vi "SR430.ProcEvents.vi"(0 "i ref in":refnum<vi>, 5 "error in (no error)":errorcluster) -> (14 "i ref out":refnum<vi>, 19 "error out":errorcluster)   [LabVIEW 2014, in "SR430.lvlib"]
doc: "Definition of commands for this class."
uses:
  SR430.lvlib
  CSCore/BaseProcess/BaseProcess.event definition.ctl
  CSCore/CAEObj/CAEObj.event definition.ctl
  CSCore/BaseProcess/BaseProcess.descriptor string definition.ctl
  CSCore/BaseProcess/BaseProcess.lvlib
  CSCore/CAEObj/CAEObj.lvlib
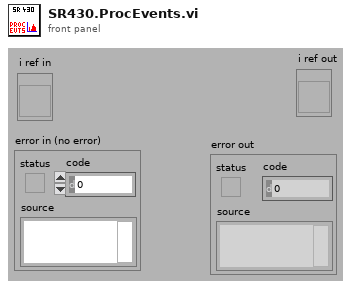
[diagram p1: front panel]
types:
  T1 = typedef "BaseProcess.lvlib/BaseProcess.event definition.ctl" = cluster{"CAEEvtDef":T2, "Data Descriptor":T3}
  T2 = typedef "CAEObj.lvlib/CAEObj.event definition.ctl" = cluster{"URL":string, "enable":bool, "ignoreResID":bool}
  T3 = typedef "BaseProcess.lvlib/BaseProcess.descriptor string definition.ctl" = string
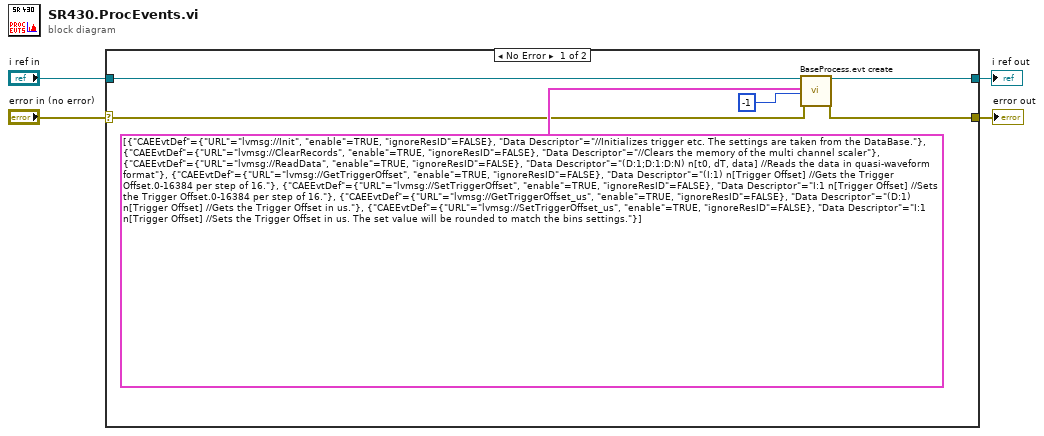
[diagram p0: block diagram]
diagram:
  n1 = case shown="No Error" "error in (no error)" {
    selector: "error in (no error)" -> [w6 w11]
    tunnel: "i ref in" -> [w10 w12]
    tunnel: [w9 w12] -> w3
    tunnel: [w8 w11] -> w2
    frame No Error {
      n2 = call "BaseProcess.evt create.vi"("i ref in"=w10, "newEvents"=T1[] [{"CAEEvtDef"={"URL"="lvmsg://Init", "enable"=TRUE, "ignoreResID"=FALSE}, "Data Descriptor"="//Initializes trigger etc. The settings are taken from the DataBase."}, {"CAEEvtDef"={"URL"="lvmsg://ClearRecords", "enable"=TRUE, "ignoreResID"=FALSE}, "Data Descriptor"="//Clears the memory of the multi channel scaler"}, {"CAEEvtDef"={"URL"="lvmsg://ReadData", "enable"=TRUE, "ignoreResID"=FALSE}, "Data Descriptor"="(D:1;D:1:D:N) n[t0, dT, data] //Reads the data in quasi-waveform format"}, {"CAEEvtDef"={"URL"="lvmsg://GetTriggerOffset", "enable"=TRUE, "ignoreResID"=FALSE}, "Data Descriptor"="(I:1) n[Trigger Offset] //Gets the Trigger Offset.0-16384 per step of 16."}, {"CAEEvtDef"={"URL"="lvmsg://SetTriggerOffset", "enable"=TRUE, "ignoreResID"=FALSE}, "Data Descriptor"="I:1 n[Trigger Offset] //Sets the Trigger Offset.0-16384 per step of 16."}, {"CAEEvtDef"={"URL"="lvmsg://GetTriggerOffset_us", "enable"=TRUE, "ignoreResID"=FALSE}, "Data Descriptor"="(D:1) n[Trigger Offset] //Gets the Trigger Offset in us."}, {"CAEEvtDef"={"URL"="lvmsg://SetTriggerOffset_us", "enable"=TRUE, "ignoreResID"=FALSE}, "Data Descriptor"="I:1 n[Trigger Offset] //Sets the Trigger Offset in us. The set value will be rounded to match the bins settings."}] ("new events"), "ms timeout (10000)"=-1, "error in (no error)"=w6) -> ("i ref out"=w9:refnum<vi>, "error out"=w8:errorcluster)  [unwired: 12 in, 2 out]
    }
    frame Error {
    }
  }
  "i ref out" <- w3
  "error out" <- w2
